vi "I2C.vi"() -> ()   [LabVIEW 2019]
uses:
  <vilib>/rvi/Emulation/niFpgaGetClockAttributes.vi
  <vilib>/rvi/Emulation/niFpgaSctlEmulationGetInTimedLoop.vi
  <vilib>/rvi/Emulation/niFpgaEmulationReportErrorSimple.vi
  <vilib>/rvi/eio/common/nirviEmuTemplateMethod_errors.vi
  <vilib>/rvi/Emulation/niFpgaCriticalErrorInLSC.vi
  <vilib>/eio/EIONode/EIONode.xnode
panel:
  out "Numeric":i32
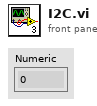
[diagram p1: front panel]
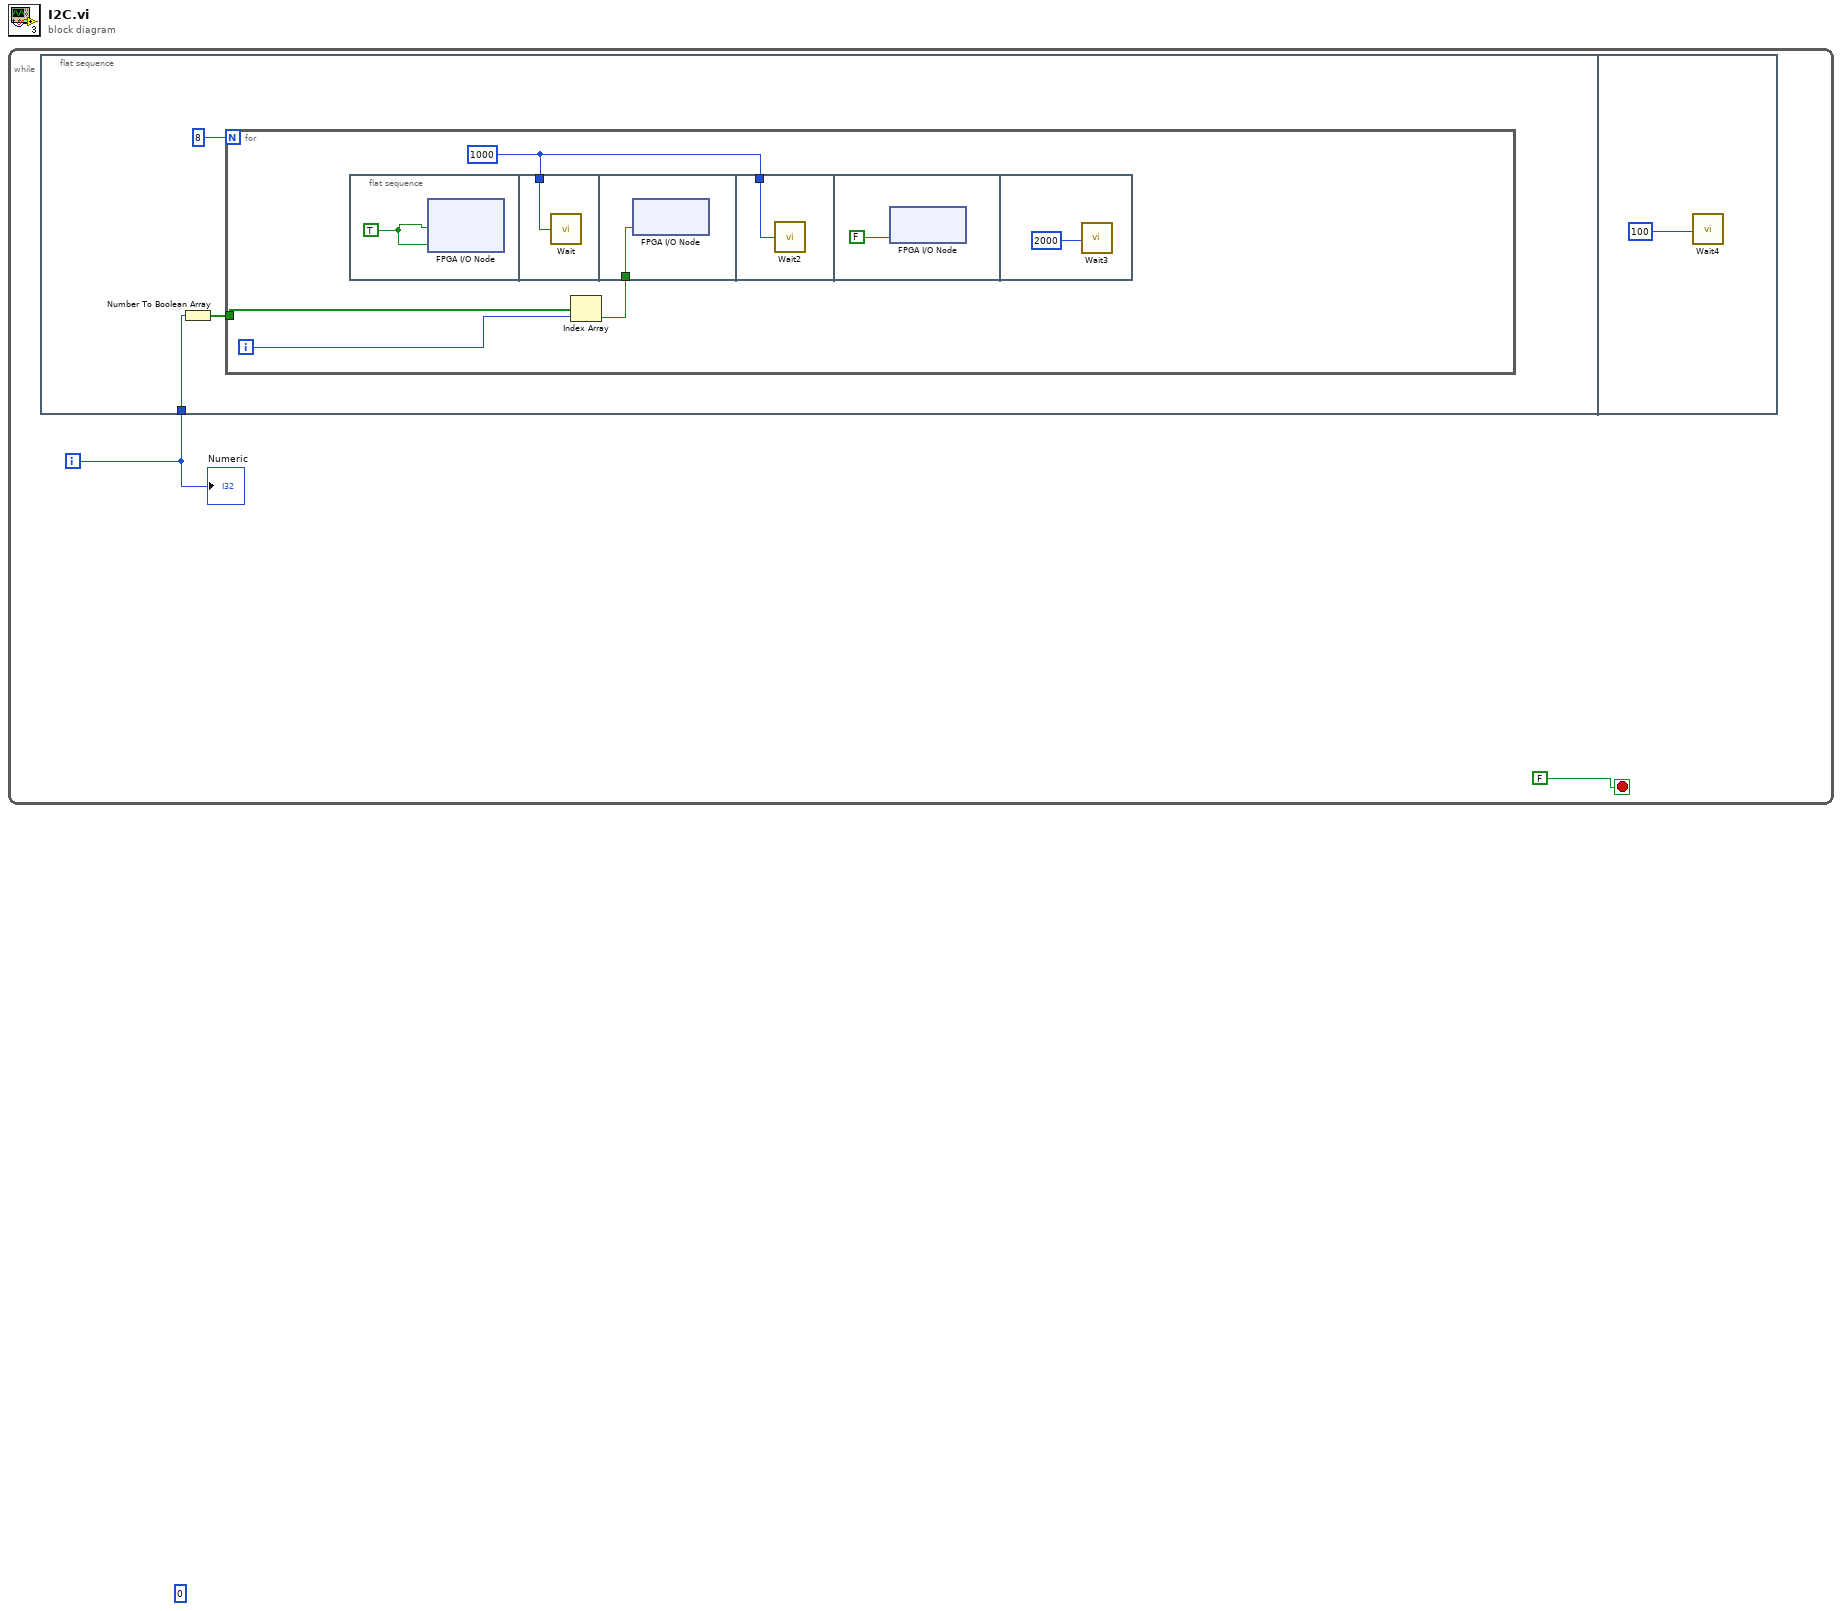
[diagram p0: block diagram]
diagram:
  (unwired) u8 0
  n1 = while {
    i -> [w1]
    stop <- FALSE stop-if-true
    n2 = flat-sequence {
      tunnel: w1 -> [w4]
      frame #0 {
        n3 = Number To Boolean Array(number=w4) -> (Boolean array=w5:bool[])
        n4 = for {
          N: u8 8 -> [_]
          tunnel: w5 -> [w6]
          i -> [w7]
          w9 = u16 1000 ("Count(Ticks)")
          n5 = flat-sequence {
            tunnel: w9 -> [w11]
            tunnel: w8 -> [w12]
            tunnel: w9 -> [w13]
            frame #0 {
              w10 = TRUE
              n6 = xnode "FPGA I/O Node"("SCL2"=w10, "SDA2"=w10) -> ()  [unwired: 2 in, 2 out]
            }
            frame #1 {
              n7 = call "Wait"("Count(Ticks)"=w11) -> ()  [unwired: 1 out]
            }
            frame #2 {
              n8 = xnode "FPGA I/O Node"("SDA2"=w12) -> ()  [unwired: 1 in, 1 out]
            }
            frame #3 {
              n9 = call "Wait2"("Count(Ticks)"=w13) -> ()  [unwired: 1 out]
            }
            frame #4 {
              n10 = xnode "FPGA I/O Node"("SCL2"=FALSE) -> ()  [unwired: 1 in, 1 out]
            }
            frame #5 {
              n11 = call "Wait3"("Count(Ticks)"=u16 2000) -> ()  [unwired: 1 out]
            }
          }
          n12 = Index Array(array=w6, index=w7) -> (element=w8:bool)
        }
      }
      frame #1 {
        n13 = call "Wait4"("Count(mSec)"=u16 100 ("Count(Ticks)")) -> ()  [unwired: 1 out]
      }
    }
    "Numeric" <- w1
  }
